vi "Snake on Food.vi"(8 "error in (no error)":errorcluster, 10 "Food Locations":refnum<class "Food.lvclass">[](array[class]), 11 "Snake in":refnum<class "Snake.lvclass">) -> (0 "error out":errorcluster, 1 "Food Index":i32, 2 "On Food?":bool, 3 "Snake out":refnum<class "Snake.lvclass">)   [LabVIEW 2020, in "Snake.lvclass"]
uses:
  Snake.lvclass
  Food/Food.lvclass
  Snake.lvclass/Snake.ctl
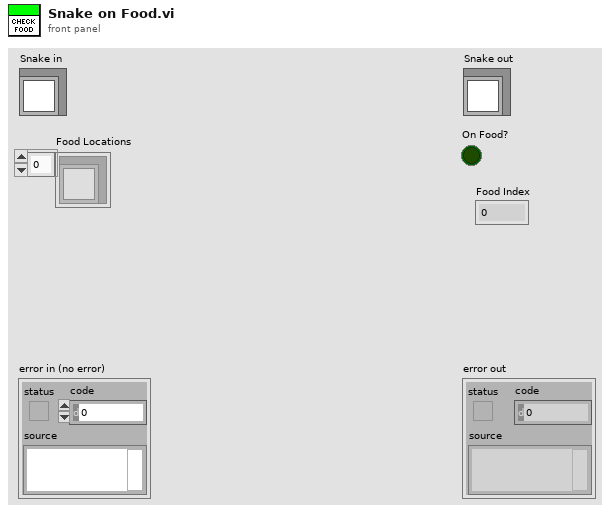
[diagram p1: front panel]
types:
  T1 = typedef "Snake.lvclass/Snake Segment STYP.ctl" = cluster{"Location":cluster{"x":u32, "y":u32}, "Direction":T2}
  T2 = typedef "Direction STYP.ctl" = enum16{"Up", "Down", "Left", "Right"}
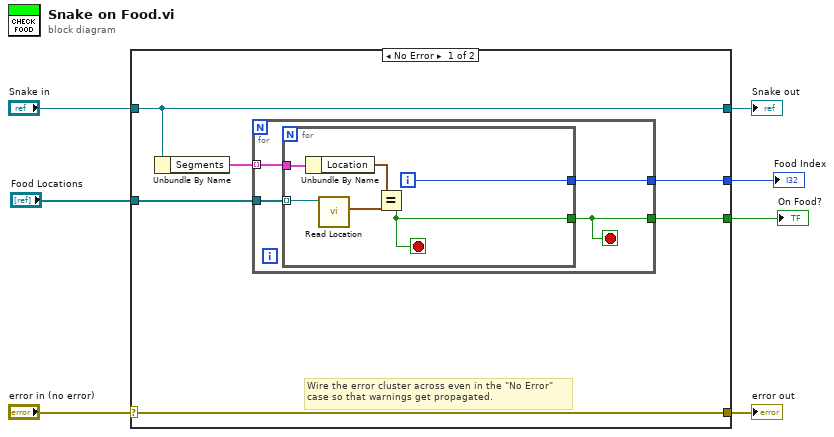
[diagram p0: block diagram]
diagram:
  n1 = case shown="No Error" "error in (no error)" {
    selector: "error in (no error)" -> [w13 w25]
    tunnel: [w13 w25] -> w6
    tunnel: [w12 w24] -> w4
    tunnel: "Snake in" -> [w12 w24]
    tunnel: "Food Locations" -> [w10 _]
    tunnel: [w9 _] -> w2
    tunnel: [w8 _] -> w1
    frame No Error {
      # "Wire the error cluster across even in the \"No Error\"\ncase so that warnings get propagated."
      n2 = Unbundle By Name(w12) -> ("Segments"=w11:T1[])
      n3 = for {
        tunnel: w11 -> [w17] mode=indexing
        tunnel: w10 -> [w16]
        tunnel: [w15] -> w8
        tunnel: [w14] -> w9
        stop <- w14 stop-if-true
        n4 = for {
          tunnel: w17 -> [w23]
          tunnel: w16 -> [w22] mode=indexing
          tunnel: [w19] -> w15
          tunnel: [w18] -> w14
          i -> [w19]
          stop <- w18 stop-if-true
          n5 = Unbundle By Name(w23) -> ("Location"=w21:cluster{"x":u32, "y":u32})
          n6 = call-dynamic "Read Location.vi"("Food in"=w22) -> ("Location"=w20:cluster{"x":u32, "y":u32})  [unwired: 8 in, 2 out]
          n7 = Equal?(x=w21, y=w20) -> (x = y?=w18:bool)
        }
      }
    }
    frame Error {
    }
  }
  "error out" <- w6
  "Snake out" <- w4
  "Food Index" <- w1
  "On Food?" <- w2
